vi "sv_Resample Engine (Angle to Time).vi"(5 "reset? (True)":bool=TRUE, 8 "error in (no error)":errorcluster, 9 "filter prototype":T2={"left wing"=[], "increment"=[], "max dec"=128, "timing jitter"=enum."Interpolation", "band limiting?"=TRUE} {"increment" format="%.2f"; "left wing" format="%.2f"}, 10 "time":dbl[](array[numeric]) format="%.2f", 11 "scaled signals (EU)":waveform(dbl)[](array[waveform])) -> (0 "error out":errorcluster, 1 "offset":dbl, 2 "time stamps":dbl[](array[numeric]) format="%.2f", 3 "Y":dbl[][](array[numeric]) format="%.2f")   [LabVIEW 2017, in "SoundVib_ContSweptSine.lvlib"]
doc: "Perform an arbitrary resampling on the input signal."
uses:
  <vilib>/addons/Sound and Vibration/svt_Continuous Swept Sine/SoundVib_ContSweptSine.lvlib
  <vilib>/addons/_NISVFA/_Shared subVIs/Controls/OAT Resample Filter Prototype.ctl
  <vilib>/addons/Sound and Vibration/Order Analysis/Resample Order Tracking/SoundVib_Resampling.lvlib
  <resource>/sndvib.dll
panel:
  in  "state in":T1 {"time interval" format="%.2f"; "position" format="%.2f"; "init condition" format="%.2f"}
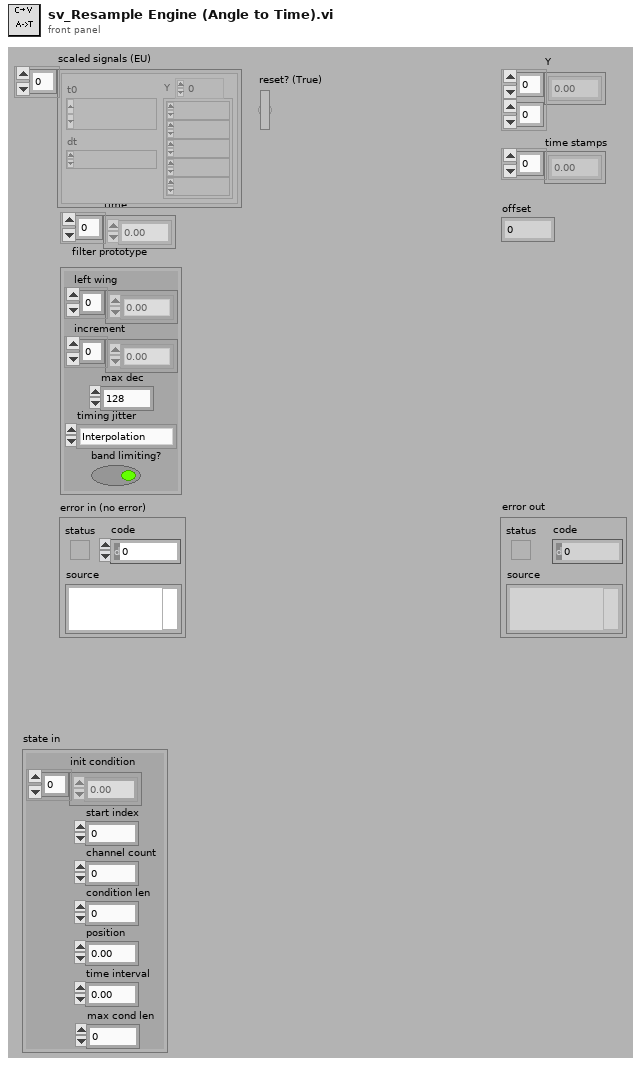
[diagram p1: front panel]
types:
  T1 = cluster{"init condition":dbl[], "start index":i32, "channel count":i32, "condition len":i32, "position":dbl, "time interval":dbl, "max cond len":i32}
  T2 = typedef "OAT Resample Filter Prototype.ctl" = cluster{"left wing":dbl[], "increment":dbl[], "max dec":i32, "timing jitter":enum32{"Interpolation", "Rounding"}, "band limiting?":bool}
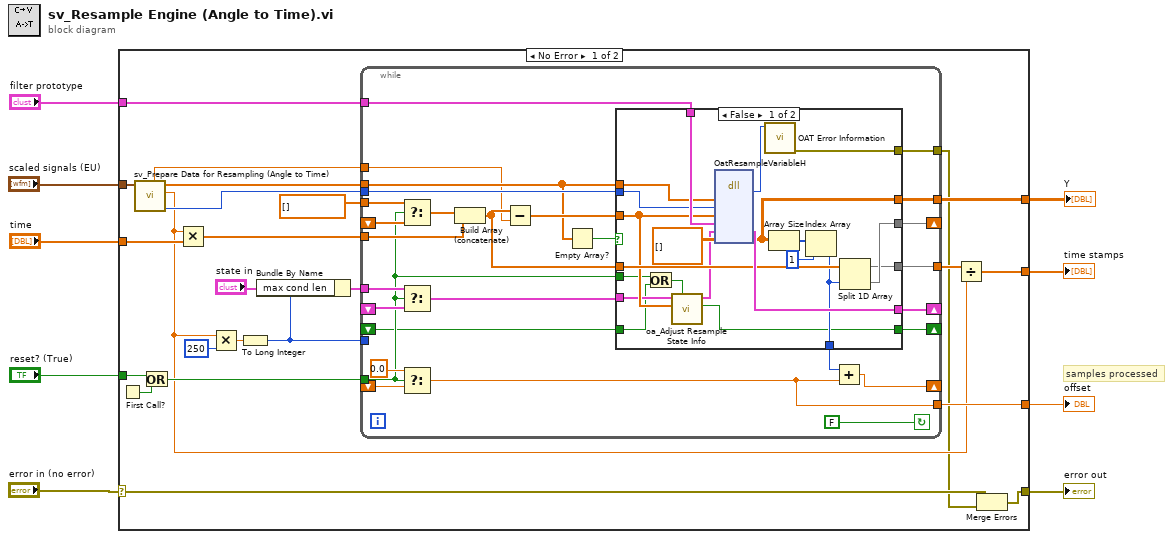
[diagram p0: block diagram]
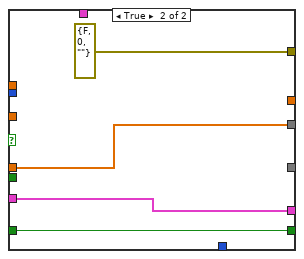
[diagram p2: hidden frame]
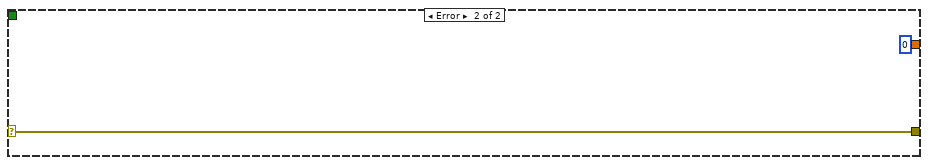
[diagram p3: hidden frame]
diagram:
  # "samples processed"
  n1 = case shown="No Error" "error in (no error)" {
    selector: "error in (no error)" -> [w13 w88]
    tunnel: "filter prototype" -> [w33 _]
    tunnel: "time" -> [w32 _]
    tunnel: [w29 _] -> w7
    tunnel: [w27 0] -> w6
    tunnel: [w11 w88] -> w5
    tunnel: "scaled signals (EU)" -> [w30 _]
    tunnel: [w24 _] -> w2
    tunnel: "reset? (True)" -> [w21 _]
    frame No Error {
      n2 = First Call?() -> (First Call?: T/F=w22:bool)
      n3 = call <vilib>:"sv_Prepare Data for Resampling (Angle to Time).vi"("Array"=w30) -> ("channel count"=w25:i32, "fs"=w19:dbl, "Y"=w31:dbl[], "elapsed length"=w10:dbl)  [unwired: 6 in, 1 out]
      n4 = Or(x=w21, y=w22) -> (x .or. y?=w20:bool)
      n5 = Multiply(x=w19, y=w32) -> (x*y=w23:dbl[])
      n6 = Multiply(x=w19, y=250) -> (x*y=w17:dbl)
      n7 = To Long Integer(number=w17) -> (32bit integer=w15:i32)
      n8 = Bundle By Name(cluster="state in", "max cond len"=w15) -> (w14:T1)
      n9 = while {
        shift-right: [w47] -> _
        shift-left: _ -> [w56]
        tunnel: w31 -> [w39]
        tunnel: w23 -> [w58]
        shift-right: [w54] -> _
        shift-left: _ -> [w59]
        tunnel: w20 -> [w41]
        tunnel: w33 -> [w48]
        shift-right: [w50] -> _
        shift-left: _ -> [w52]
        tunnel: [w60] -> w12
        tunnel: [w40] -> w29
        tunnel: w14 -> [w57]
        tunnel: dbl[] [] ("t") -> [w53]
        tunnel: [w45] -> w26
        tunnel: [w49] -> w27
        tunnel: w25 -> [w46]
        tunnel: w15 -> [_]
        tunnel: w10 -> [w38]
        shift-right: [w35] -> _
        shift-left: _ -> [w34]
        stop <- FALSE continue-if-true
        n10 = Select(t=w53, s=w41, f=w59) -> (s? t:f=w55:dbl[])
        n11 = Select(t=w57, s=w41, f=w56) -> (s? t:f=w37:T1)
        n12 = Select(t=0.0, s=w41, f=w52) -> (s? t:f=w49:dbl)
        n13 = Build Array (concatenate)(w55, w58) -> (w44:dbl[])
        n14 = Subtract(x=w44, y=w38) -> (x-y=w42:dbl[])
        n15 = Empty Array?(array=w39) -> (empty?=w36:bool)
        n16 = case shown="False" w36 {
          tunnel: [w82 errorcluster {"status"=FALSE, "code"=0, "source"=""} ("error out")] -> w60
          tunnel: [w81 w86] -> w54
          tunnel: w48 -> [w80 _]
          tunnel: [w79 w85] -> w47
          tunnel: w46 -> [w78 _]
          tunnel: [w77 _] -> w45
          tunnel: w44 -> [w76 w86]
          tunnel: [w75 _] -> w43
          tunnel: w42 -> [w74 _]
          tunnel: w41 -> [w64 _]
          tunnel: [w73 _] -> w40
          tunnel: w39 -> [w72 _]
          tunnel: w37 -> [w71 w85]
          tunnel: [w65 w83] -> w35
          tunnel: w34 -> [w63 w83]
          frame False {
            n17 = Or(x=w64, y=w63) -> (x .or. y?=w62:bool)
            n18 = call <vilib>:"oa_Adjust Resample State Info.vi"("Reset? (True)"=w62, "time position"=w74, "state in"=w71) -> ("reset pending"=w65:bool, "state out"=w66:T1)  [unwired: 1 in, 6 out]
            n19 = dll-call lib="C:/Program Files (x86)/National Instruments/LabVIEW 2017/resource/sndvib.*" fn="OatResampleVariableH"("signalH"=w72, "channelCount"=w78, "timeH"=w74, "prototype"=w80, "state"=w66, "yH"=dbl[][] []) -> ("return type"=w70:i32, "state"=w79:T1, "yH"=w73:dbl[][])  [unwired: 7 in, 2 out]
            n20 = call <vilib>:"OAT Error Information.vi"("error code"=w70) -> ("error out"=w82:errorcluster)  [unwired: 6 in]
            n21 = Array Size(array=w73) -> (size(s)=w68:i32[])
            n22 = Index Array(array=w68, index=1) -> (element=w75:i32)
            n23 = Split 1D Array(array=w76, index=w75) -> (first subarray=w77:dbl[], second subarray=w81:dbl[])
          }
          frame True {
          }
        }
        n24 = Add(x=w43, y=w49) -> (x+y=w50:dbl)
      }
      n25 = Divide(x=w26, y=w19) -> (x/y=w24:dbl[])
      n26 = Merge Errors(w13, w12) -> (w11:errorcluster)
    }
    frame Error {
    }
  }
  "time stamps" <- w2
  "Y" <- w7
  "offset" <- w6
  "error out" <- w5
